vi "Configure IQ Recorder Measurement Timeout.vi"(8 "error in (no error)":errorcluster, 9 "Measurement Timeout (1)":dbl=1.0 format="%^.3e", 10 "Instance (1)":i32=1, 11 "VISA resource name":refnum<visa-resource-name>) -> (0 "error out":errorcluster, 3 "VISA resource name out":refnum<visa-resource-name>)   [LabVIEW 2015, in "Rohde&Schwarz CMXP GPRF.lvlib"]
doc: "Defines a timeout for the measurement. The timer is started when the measurement is initiated via a READ or INIT command. It is not started if the measurement is initiated manually ([ON | OFF] key or [RESTART | STOP] key).When the measurement has completed the first measurement cycle (first single shot), the statistical depth is reached and the timer is reset.If the first measurement cycle has not been completed when the timer expires, the measurement is stopped. The measurement state changes to RDY. The reliability indicator is set to 1, indicating that a measurement timeout occurred. Still running READ, FETCh or CALCulate commands are completed, returning the available results. At least for some results, there are no values at all or the statistical depth has not been reached.A timeout of 0 s corresponds to an infinite measurement timeout.\n\nAttribute:\nRSCMXPGPRF_ATTR_IQ_RECORDER_MEASUREMENT_TIMEOUT\n\nRemote-control command:\nCONFigure:GPRF:MEAS<i>:IQRecorder:TOUT"
uses:
  <instrlib>/Rohde&Schwarz CMXP GPRF/Rohde&Schwarz CMXP GPRF.lvlib
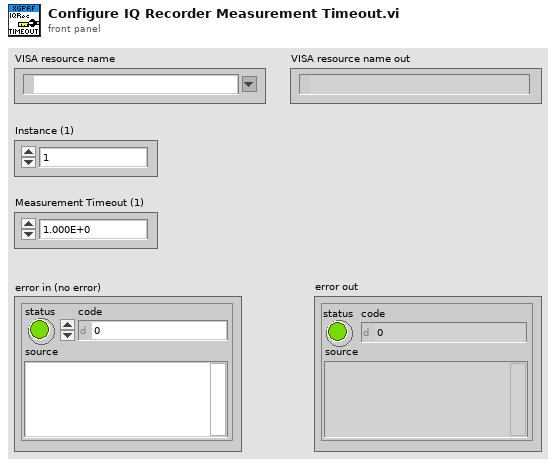
[diagram p1: front panel]
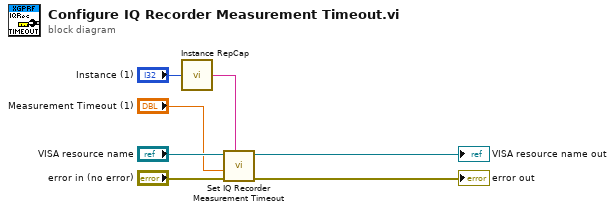
[diagram p0: block diagram]
diagram:
  n1 = call <instrlib>:"Instance RepCap.vi"("instance  in"="Instance (1)") -> ("instance out"=w2:string)
  n2 = call "Set IQ Recorder Measurement Timeout"("Repeated Capabilities"=w2, "error in (no error)"="error in (no error)", "IQ Recorder Measurement Timeout (0.0)"="Measurement Timeout (1)", "instrument handle"="VISA resource name") -> ("error out"=→"error out":errorcluster, "instrument handle out"=→"VISA resource name out":refnum<visa-resource-name>)  [unwired: 6 in]
